vi "Display Console.vi"(8 "error in (no error)":errorcluster) -> (0 "error out":errorcluster)   [LabVIEW 2017]
uses:
  Type Definitions/Queue FG Options.ctl
panel:
  out "Card Read":bool
  out "Message Screen":string
  out "Current Transaction":string
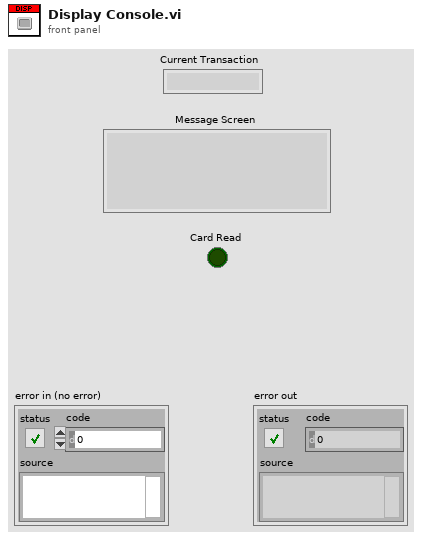
[diagram p1: front panel]
types:
  T1 = typedef "Queue FG Options.ctl" = enum16{"Set", "Get", "Read", "Write"}
  T2 = typedef "Message.ctl" = cluster{"Message Info":string, "Message Data":variant}
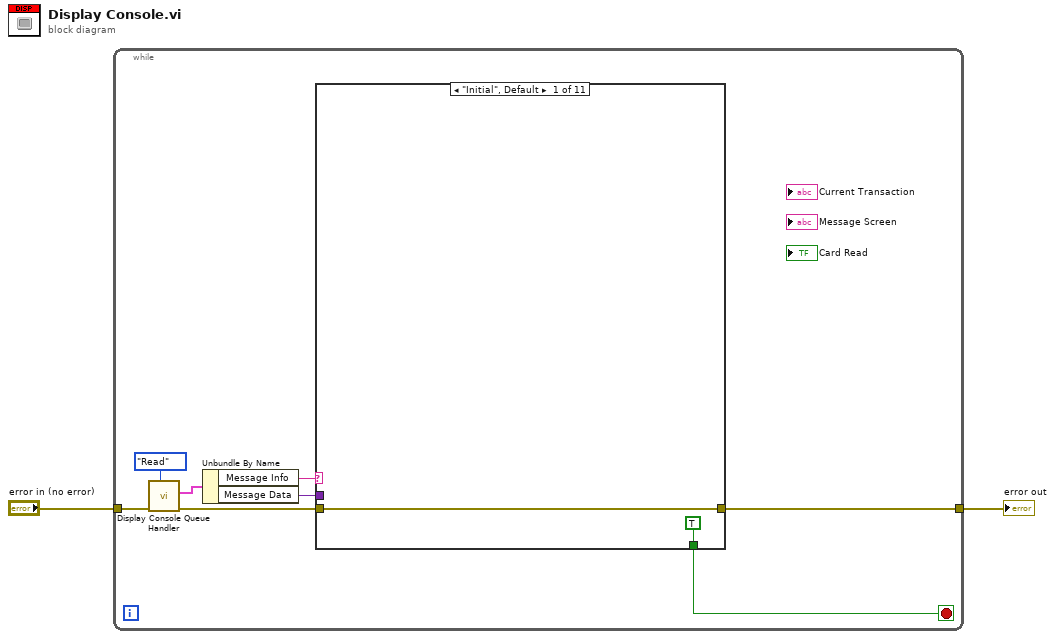
[diagram p0: block diagram]
diagram:
  n1 = while {
    tunnel: "error in (no error)" -> [w9]
    tunnel: [w4] -> w1
    stop <- w3 stop-if-true
    n2 = call "Display Console Queue Handler.vi"("Action"=Queue_FG_Options."Read", "error in (no error)"=w9) -> ("error out"=w5:errorcluster, "Message out"=w8:T2)  [unwired: 7 in, 1 out]
    n3 = Unbundle By Name(w8) -> ("Message Info"=w7:string, "Message Data"=w6:variant)
    n4 = case shown="\"Initial\", Default" w7 {
      tunnel: w6 -> [_ _ _ _ _ _ _ _ _ _ _]
      tunnel: w5 -> [w12 w13 w14 w15 w16 w17 w18 w19 w20 w21 w22]
      tunnel: [w12 w13 w14 w15 w16 w17 w18 w19 w20 w21 w22] -> w4
      tunnel: [TRUE _ _ _ _ _ _ _ _ _ _] -> w3
      frame "Initial", Default {
      }
      frame "Login" {
      }
      frame "Invalid Login" {
      }
      frame "Idle " {
      }
      frame "Balance Inquiry" {
      }
      frame "Deposit" {
      }
      frame "Withdrawal" {
      }
      frame "Fast Cash" {
      }
      frame "Withdrawal Failed" {
      }
      frame "Withdrawal Complete" {
      }
      frame "Terminate" {
      }
    }
  }
  "error out" <- w1
